vi "SetChannel(Vertical).vi"(8 "error in (no error)":errorcluster, 11 "TektronixDPO in":refnum<class "TektronixDPO.lvclass">) -> (0 "error out":errorcluster, 3 "TektronixDPO Out":refnum<class "TektronixDPO.lvclass">)   [LabVIEW 2013, in "TektronixDPO.lvclass"]
doc: "Send the channel settings to the physical device and read them back"
uses:
  TektronixDPO.lvclass
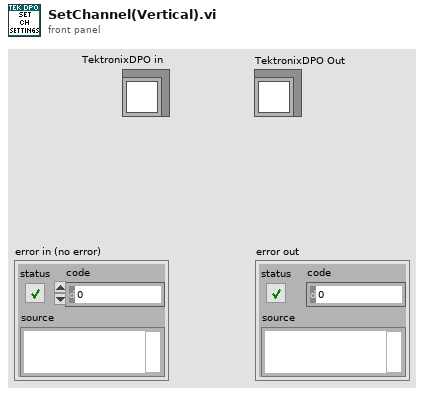
[diagram p1: front panel]
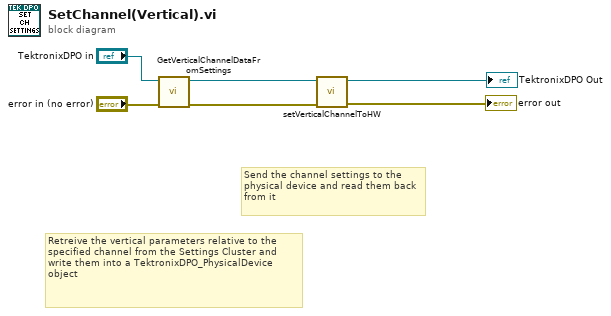
[diagram p0: block diagram]
diagram:
  # "Retreive the vertical parameters relative to the specified channel from the Settings Cluster and write them into a TektronixDPO_PhysicalDevice object"
  # "Send the channel settings to the physical device and read them back from it"
  n1 = call "GetVerticalChannelDataFromSettings.vi"("error in (no error)"="error in (no error)", "TektronixDPO in"="TektronixDPO in") -> ("error out"=w6:errorcluster, "TektronixDPO Out"=w5:refnum<class "TektronixDPO.lvclass">)  [unwired: 8 in]
  n2 = call "setVerticalChannelToHW.vi"("error in (no error)"=w6, "TektronixDPO in"=w5) -> ("error out"=→"error out":errorcluster, "TektronixDPO out"=→"TektronixDPO Out":refnum<class "TektronixDPO.lvclass">)  [unwired: 8 in]
